vi "Dynamic1DArray.vi"() -> ()   [LabVIEW 2020]
uses:
  Passing.dll
panel:
  in  "size":i32=5
  out "arg1 2":dbl[](array[numeric])=[5.29462817e-315, 5.30239915e-315, 5.30628464e-315, 5.30887497e-315, -3.744075715666969e-103]
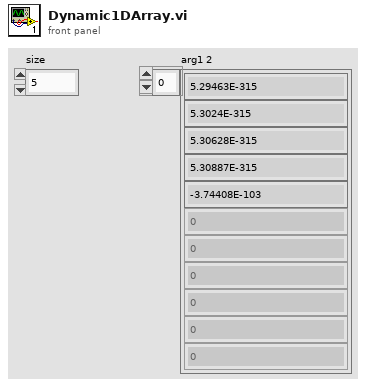
[diagram p1: front panel]
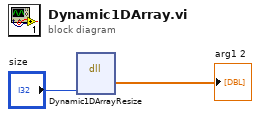
[diagram p0: block diagram]
diagram:
  n1 = dll-call lib="E:/Practice/Lv/dll/CppDllForLv/src/LV/Passing/Passing.dll" fn="Dynamic1DArrayResize"("size"="size") -> ("arg1"=→"arg1 2":dbl[])  [unwired: 6 in, 2 out]
